vi "PPL_ActionVIOnCompile_InlineAsync.vi"(8 "error in (no error)":errorcluster, 11 "Device Item Ref in":T1 format="%.0x") -> (0 "error out":errorcluster)   [LabVIEW 2019]
uses:
  <vilib>/NI VeriStand/Custom Device API/Custom Device Item Ref.ctl
  <vilib>/NI VeriStand/Custom Device API/Get Item Property (U16).vi
  <vilib>/NI VeriStand/Custom Device Tools/Custom Device Utility Library/NI VeriStand - Search for Item by Name.vi
  <vilib>/NI VeriStand/Custom Device API/Set Item Property (Variant).vi
  <vilib>/NI VeriStand/Custom Device Tools/Custom Device Utility Library/Custom Device Utility Library.lvlib
  <vilib>/NI VeriStand/Custom Device API/Custom Device API.lvlib
  <vilib>/NI/NIVS Inline Async API/_Data Access System Explorer/Data Access System Explorer.lvlib
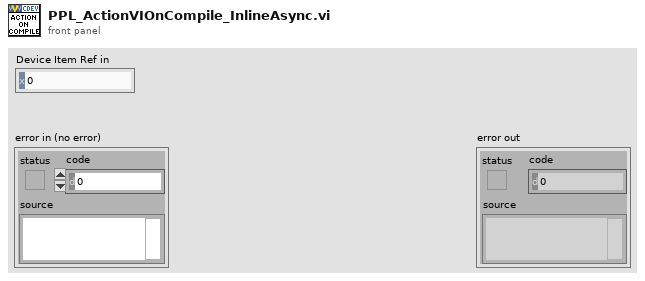
[diagram p1: front panel]
types:
  T1 = typedef "Custom Device API.lvlib/Custom Device Item Ref.ctl" = u64
  T2 = cluster{"Name":string, "Type":enum16{"Output/Write", "Input/Read", "Input/ReadWrite"}, "VS Refs":T1[]}
  T3 = enum16{"Output/Write", "Input/Read", "Input/ReadWrite"}
  T4 = typedef "Custom Device API.lvlib/Custom Device Item Info.ctl" = cluster{"Name":string, "Is Channel":bool, "GUID":string, "Is Waveform":bool}
  T5 = cluster{"Name":string, "Type":enum16{"Output/Write", "Input/Read", "Input/ReadWrite"}, "VS Refs":T1[]}[]
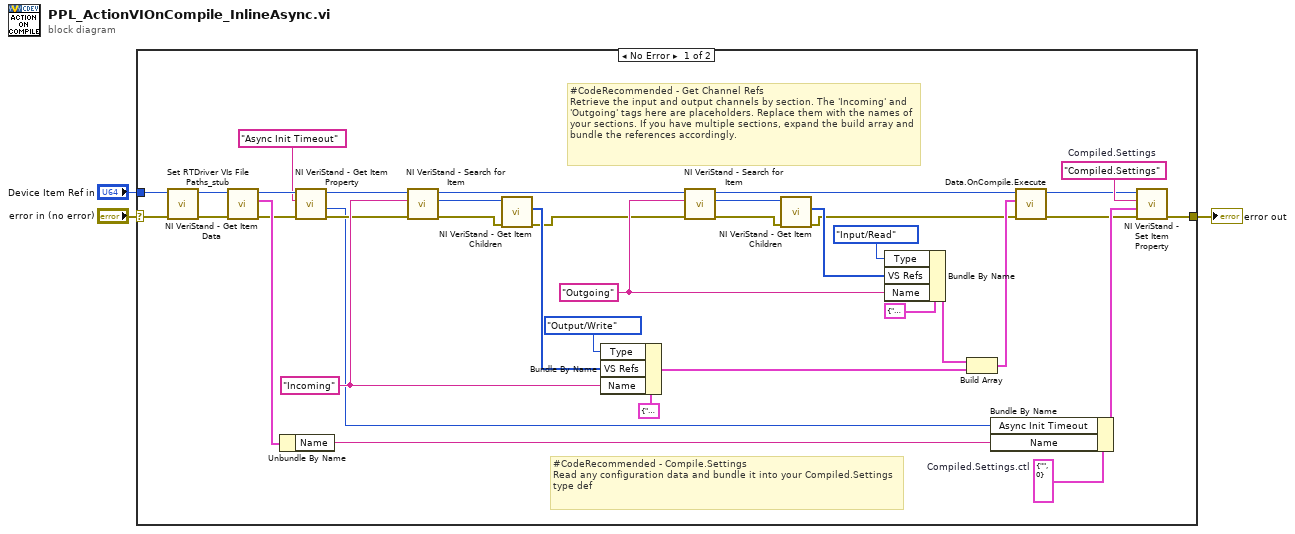
[diagram p0: block diagram]
diagram:
  n1 = case shown="No Error" "error in (no error)" {
    selector: "error in (no error)" -> [w6 w41]
    tunnel: [w34 w41] -> w2
    tunnel: "Device Item Ref in" -> [w7 _]
    frame No Error {
      w14 = cluster{"Name":string, "Async Init Timeout":u16} {"Name"="", "Async Init Timeout"=0}  # Compiled.Settings.ctl
      w29 = "Outgoing" ("Item Name")
      w31 = "Incoming" ("Item Name")
      w36 = "Compiled.Settings"  # Compiled.Settings
      # "#CodeRecommended - Get Channel Refs\nRetrieve the input and output channels by section. The 'Incoming' and 'Outgoing' tags here are placeholders. Replace them with the names of your sections. If you have multiple sections, expand the build array and bundle the references accordingly."
      # "#CodeRecommended - Compile.Settings\nRead any configuration data and bundle it into your Compiled.Settings type def"
      n2 = call "Set RTDriver VIs File Paths_stub.vi"("error in (no error)"=w6, "Item Ref in"=w7) -> ("error out"=w4:errorcluster, "Item Ref out"=w5:T1)  [unwired: 8 in]
      n3 = call <vilib>:"NI VeriStand - Get Item Data.vi"("error in (no error)"=w4, "Item Ref in"=w5) -> ("error out"=w13:errorcluster, "Item Info"=w33:T4, "Item Ref out"=w11:T1)  [unwired: 6 in, 1 out]
      n4 = Unbundle By Name(w33) -> ("Name"=w32:string)
      n5 = call-poly <vilib>:"NI VeriStand - Get Item Property.vi"("error in (no error)"=w13, "Property Name"="Async Init Timeout", "Item Ref in"=w11) -> ("error out"=w12:errorcluster, "Value"=w8:u16, "Item Ref out"=w10:T1)  [unwired: 5 in, 1 out]
      n6 = call-poly <vilib>:"NI VeriStand - Search for Item.vi"("error in"=w12, "Item Name"=w31, "Section Ref in"=w10) -> ("error out"=w40:errorcluster, "Item Ref"=w39:T1, "Section Ref out"=w18:T1)  [unwired: 5 in, 1 out]
      n7 = call <vilib>:"NI VeriStand - Get Item Children.vi"("error in (no error)"=w40, "Item Ref in"=w39) -> ("error out"=w17:errorcluster, "Child Refs"=w30:T1[])  [unwired: 6 in, 2 out]
      n8 = Bundle By Name(cluster=T2 {"Name"="", "Type"=enum."Output/Write", "VS Refs"=[]} ("Group"), "Type"=T3."Output/Write", "VS Refs"=w30, "Name"=w31) -> (w21:T2)
      n9 = call-poly <vilib>:"NI VeriStand - Search for Item.vi"("error in"=w17, "Item Name"=w29, "Section Ref in"=w18) -> ("error out"=w37:errorcluster, "Item Ref"=w38:T1, "Section Ref out"=w19:T1)  [unwired: 5 in, 1 out]
      n10 = call <vilib>:"NI VeriStand - Get Item Children.vi"("error in (no error)"=w37, "Item Ref in"=w38) -> ("error out"=w20:errorcluster, "Child Refs"=w25:T1[])  [unwired: 6 in, 2 out]
      n11 = Bundle By Name(cluster=T2 {"Name"="", "Type"=enum."Output/Write", "VS Refs"=[]} ("Group"), "Type"=T3."Input/Read", "VS Refs"=w25, "Name"=w29) -> (w27:T2)
      n12 = Build Array(w27, w21) -> (w24:T5)
      n13 = Bundle By Name(cluster=w14, "Async Init Timeout"=w8, "Name"=w32) -> (w35:cluster{"Name":string, "Async Init Timeout":u16})
      n14 = call <vilib>:"Data.OnCompile.Execute.vi"("error in"=w20, "VS Ref Groups"=w24, "Custom Device Ref"=w19) -> ("error out"=w16:errorcluster, "Custom Device Ref"=w15:T1)  [unwired: 7 in]
      n15 = call-poly <vilib>:"NI VeriStand - Set Item Property.vi"("error in (no error)"=w16, "Value"=w35, "Property Name"=w36, "Item Ref in"=w15) -> ("error out"=w34:errorcluster)  [unwired: 5 in, 2 out]
    }
    frame Error {
    }
  }
  "error out" <- w2
